vi "FRR_Query.vi"(0 "System no.":i32=1 min=1 max=4 step=1, 2 "Routinename":string[](array[string]), 3 "ResultID":i32[](array[numeric]), 4 "Query all?":bool, 5 "error in":errorcluster, 6 "Use FRH?":bool) -> (12 "ResultID Meaning":string[](array[string]), 13 "Value Unit":string[](array[string]), 14 "Value (num.)":dbl[](array[numeric]) format="%.6f", 15 "Value (string)":string[](array[string]), 16 "Queried routinename out":string[](array[string]), 17 "ResultID out":i32[](array[numeric]), 19 "error out":errorcluster)   [LabVIEW 2020]
doc: "Get results of given fast alignment routine. If Use FRH? is TRUE, VI queries FRH? and returns meaning of ResultIDs and units of Values. Requires FRH? and Parse_FRH_Type_String.vi.\n\nE-712, E-727.AS: Query all? must be FALSE, Use FRH? can be TRUE.\n\nC-887, E-712, E-727.AS:"
uses:
  Global1.vi
panel:
  # "Get results of given fast alignment procedure"
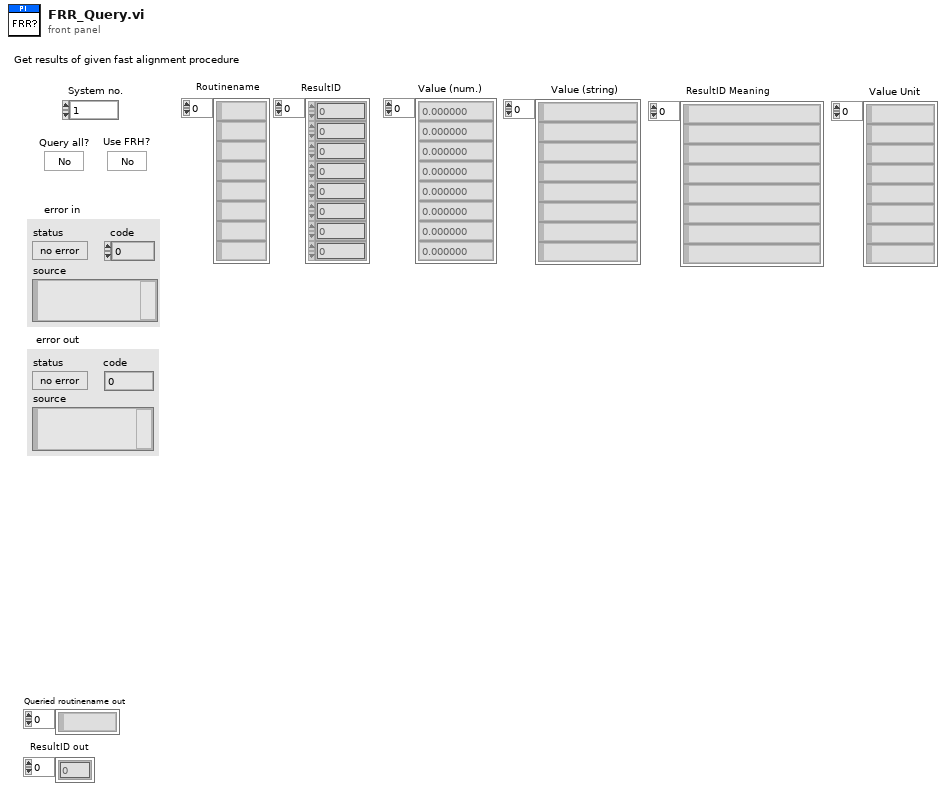
[diagram p1: front panel]
types:
  T1 = typedef "Syntax.ctl" = enum16{"GCS 1.0", "GCS 2.0", "GCS 3.0"}
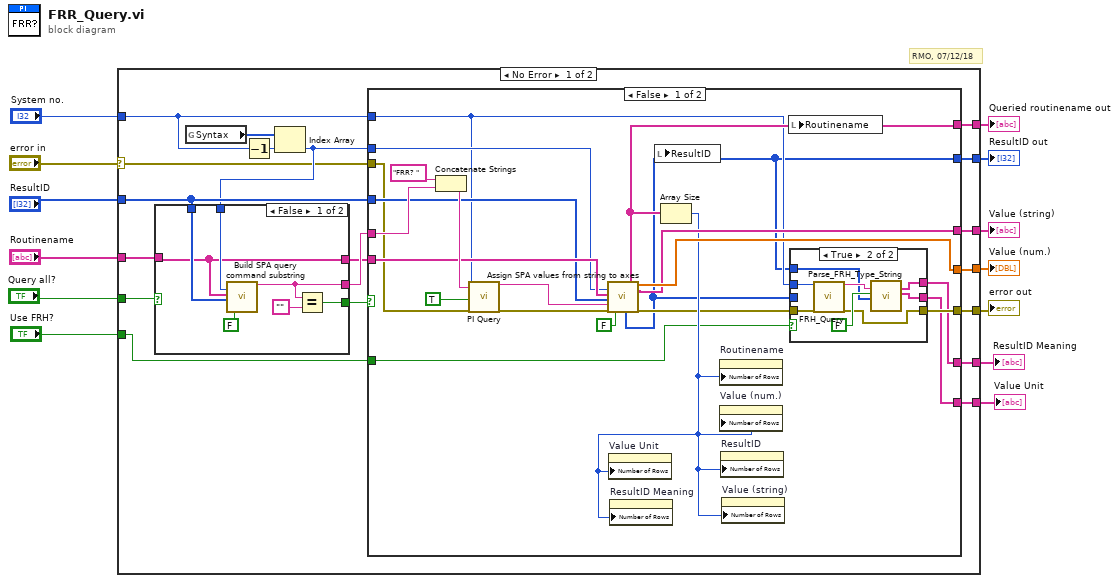
[diagram p0: block diagram]
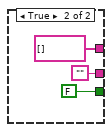
[diagram p2: hidden frame]
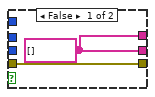
[diagram p3: hidden frame]
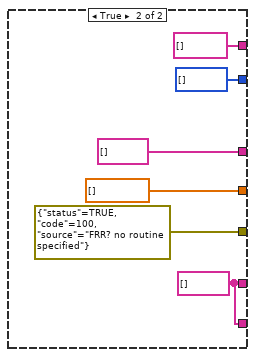
[diagram p4: hidden frame]
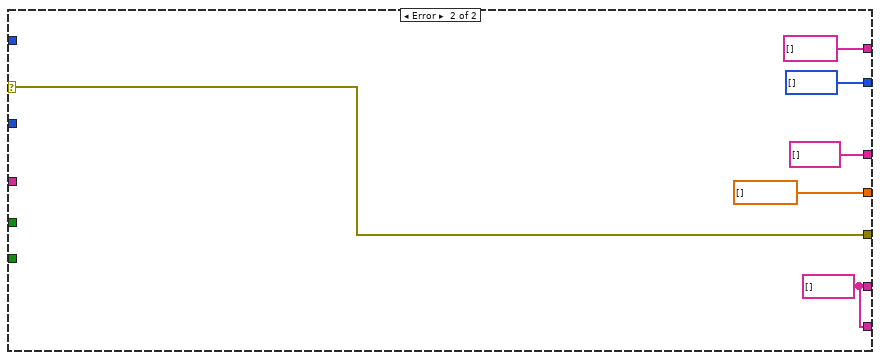
[diagram p5: hidden frame]
diagram:
  # "RMO, 07/12/18"
  n1 = case shown="No Error" "error in" {
    selector: "error in" -> [w14 w81]
    tunnel: "Routinename" -> [w32 _]
    tunnel: "System no." -> [w21 _]
    tunnel: "ResultID" -> [w29 _]
    tunnel: [w28 w81] -> w10
    tunnel: [w26 dbl[] [] ("Parameter values")] -> w9
    tunnel: "Query all?" -> [w25 _]
    tunnel: [w24 string[] [] ("Parameter strings")] -> w8
    tunnel: [w19 string[] [] ("Queried axes out")] -> w7
    tunnel: [w18 i32[] [] ("Parameter no. out")] -> w6
    tunnel: [w17 w82] -> w4
    tunnel: [w16 w82] -> w3
    tunnel: "Use FRH?" -> [w15 _]
    frame No Error {
      n2 = global read "Global1.vi" "Syntax"() -> (w22:T1[])
      n3 = Decrement(x=w21) -> (x-1=w23:i32)
      n4 = Index Array(array=w22, index=w23) -> (element=w20:T1)
      n5 = case shown="False" w25 {
        tunnel: w32 -> [w35 _]
        tunnel: [w39 "" ("Command substring")] -> w31
        tunnel: [w35 string[] [] ("Designator to query")] -> w30
        tunnel: w29 -> [w38 _]
        tunnel: [w37 FALSE] -> w27
        tunnel: w20 -> [w36 _]
        frame False {
          n6 = call "Build SPA query command substring.vi"("Syntax"=w36, "Axes to query"=w35, "Parameter number"=w38, "Parameter no. format \n(Decimal: FALSE)"=FALSE ("Parameter no. format \n(Decimal: FALSE)")) -> ("Command substring"=w39:string)  [unwired: 3 in, 12 out]
          n7 = Equal?(x=w39, y="" ("x")) -> (x = y?=w37:bool)
        }
        frame True {
        }
      }
      n8 = case shown="False" w27 {
        tunnel: w14 -> [w56 _]
        tunnel: w31 -> [w61 _]
        tunnel: w30 -> [w60 _]
        tunnel: w21 -> [w49 _]
        tunnel: w29 -> [w59 _]
        tunnel: [w50 errorcluster {"status"=TRUE, "code"=100, "source"="FRR? no routine specified"} ("error out")] -> w28
        tunnel: [w58 dbl[] [] ("Parameter values")] -> w26
        tunnel: [w57 string[] [] ("Parameter strings")] -> w24
        tunnel: w20 -> [w55 _]
        tunnel: [w54 string[] [] ("Queried axes out")] -> w19
        tunnel: [w45 i32[] [] ("Parameter no. out")] -> w18
        tunnel: [w48 w75] -> w17
        tunnel: [w47 w75] -> w16
        tunnel: w15 -> [w46 _]
        frame False {
          n9 = Concatenate Strings("FRR? ", w61) -> (w62:string)
          n10 = call "PI Query.vi"("System no."=w49, "String to send"=w62, "Attach termination char.?"=TRUE ("Attach Linefeed?"), "error in"=w56) -> ("String read"=w44:string, "error out"=w43:errorcluster)  [unwired: 3 in, 11 out]
          n11 = call "Assign SPA values from string to axes.vi"("Syntax"=w55, "Queried axes"=w60, "Parameter no."=w59, "Input string"=w44, "error in"=w43, "Parameter no. format \n(Decimal: FALSE)"=FALSE ("Parameter no. format \n(Decimal: FALSE)")) -> ("Parameter no. out"=w45:i32[], "Queried axes out"=w54:string[], "Parameter values"=w58:dbl[], "Parameter strings"=w57:string[], "error out"=w51:errorcluster)  [unwired: 2 in, 7 out]
          n12 = local write "ResultID"(w45) -> ()
          n13 = Array Size(array=w54) -> (size(s)=w52:i32)
          n14 = property on="Value Unit" class="Arr (strict)"("Number of Rows"=w52) -> ()  [unwired: 2 in, 2 out]
          n15 = property on="ResultID Meaning" class="Arr (strict)"("Number of Rows"=w52) -> ()  [unwired: 2 in, 2 out]
          n16 = property on="Routinename" class="Arr (strict)"("Number of Rows"=w52) -> ()  [unwired: 2 in, 2 out]
          n17 = property on="Value (num.)" class="Arr (strict)"("Number of Rows"=w52) -> ()  [unwired: 2 in, 2 out]
          n18 = property on="ResultID" class="Arr (strict)"("Number of Rows"=w52) -> ()  [unwired: 2 in, 2 out]
          n19 = property on="Value (string)" class="Arr (strict)"("Number of Rows"=w52) -> ()  [unwired: 2 in, 2 out]
          n20 = local write "Routinename"(w54) -> ()
          n21 = case shown="True" w46 {
            tunnel: w51 -> [w66 w74]
            tunnel: [w66 w69] -> w50
            tunnel: w49 -> [_ w73]
            tunnel: [w65 w68] -> w48
            tunnel: [w65 w67] -> w47
            tunnel: w45 -> [_ _]
            tunnel: w45 -> [_ w70]
            frame False {
              w65 = string[] [] ("Value Unit Out")
            }
            frame True {
              n22 = call "FRH_Query.vi"("System no."=w73, "error in"=w74) -> ("FRR? help string"=w72:string, "error out"=w69:errorcluster)  [unwired: 16 out]
              n23 = call "Parse_FRH_Type_String.vi"("String In"=w72, "All IDs?"=FALSE, "IDs In"=w70) -> ("String 1 Out"=w68:string[], "String 2 Out"=w67:string[])  [unwired: 15 out]
            }
          }
        }
        frame True {
          w75 = string[] [] ("Meaning Out")
        }
      }
    }
    frame Error {
      w82 = string[] [] ("Meaning Out")
    }
  }
  "error out" <- w10
  "Value (num.)" <- w9
  "Value (string)" <- w8
  "Queried routinename out" <- w7
  "ResultID out" <- w6
  "ResultID Meaning" <- w4
  "Value Unit" <- w3
